vi "RegTester.vi"() -> ()   [LabVIEW 2012]
uses:
  <vilib>/Utility/file.llb/Write To Spreadsheet File (DBL).vi
  <vilib>/vision/NI_Vision_Development_Module.lvlib
panel:
  out "alignment quality":dbl[](graph)
  out "x translation":dbl[](graph)
  in  "x translation file":path
  in  "quality array file":path
  out "error out":errorcluster
  in  "Registration parameters":T1={"Sampling Percentage"=0.2, "maximum iteration"=200, "number of bins"=200}
  in  "background":path
  in  "image folder":path
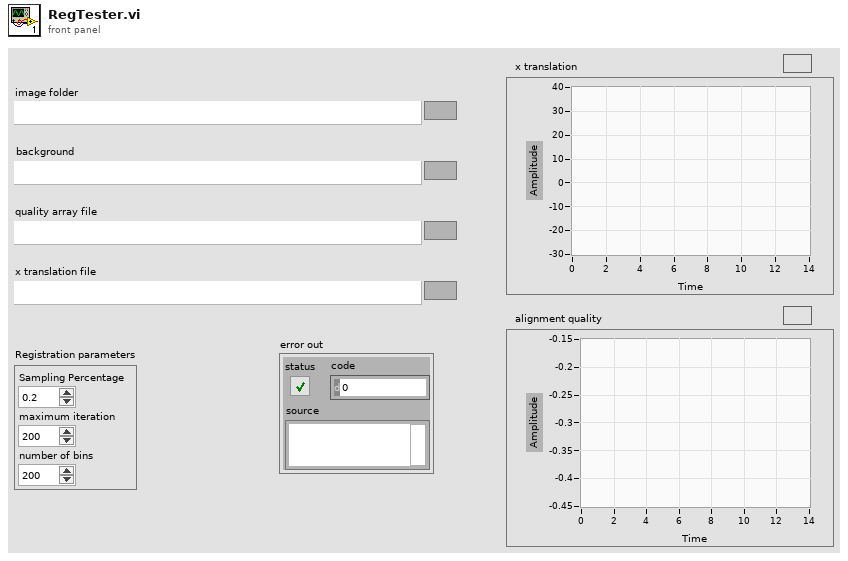
[diagram p1: front panel]
types:
  T1 = cluster{"Sampling Percentage":dbl, "maximum iteration":i32, "number of bins":u32}
  T2 = typedef "Image Type" = u32
  T3 = typedef "IMAQ Image.ctl" = refnum<image>
  T4 = typedef "ROI Descriptor" = cluster{"Global Rectangle":i32[], "Contours":cluster{"ID":enum32{"External", "Internal"}, "Type":u32, "Coordinates":i32[]}[]}
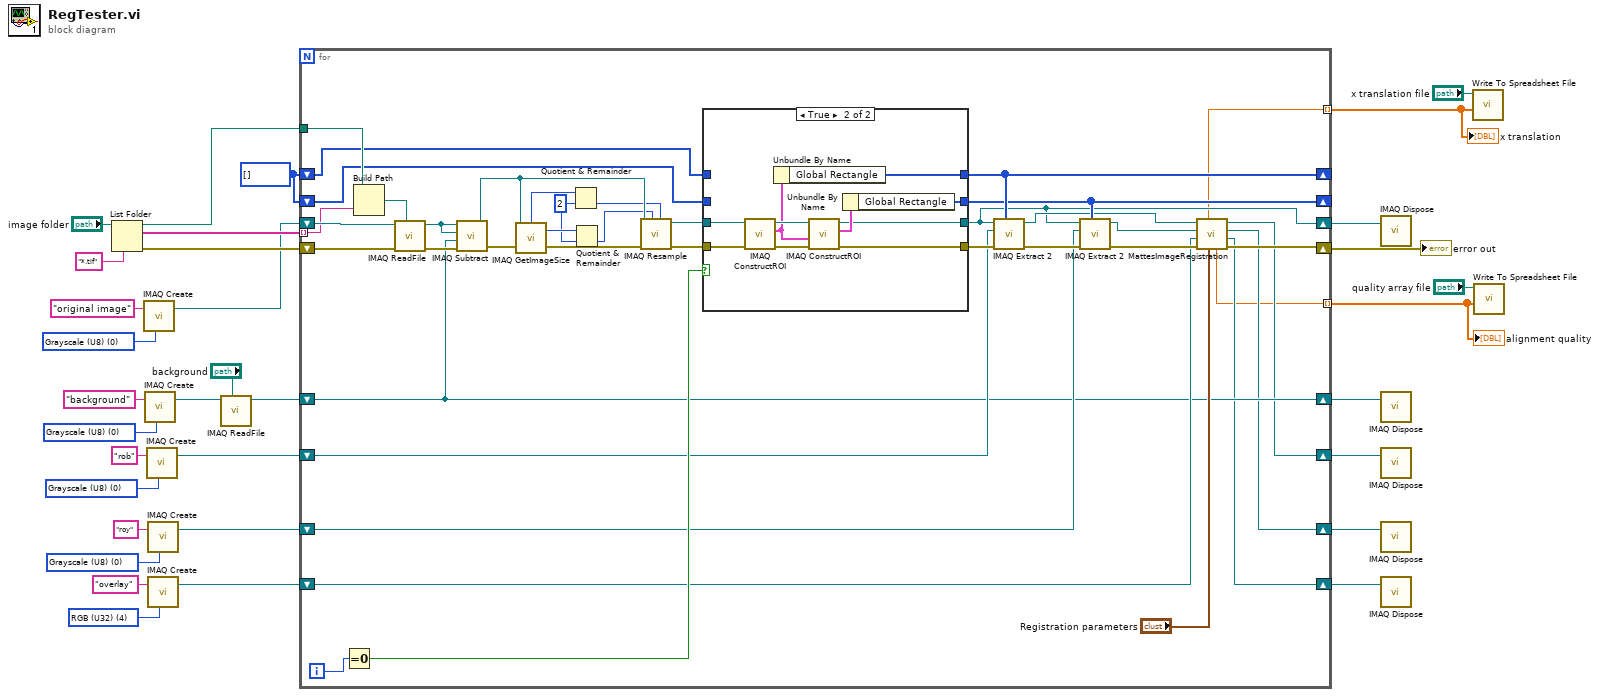
[diagram p0: block diagram]
diagram:
  w14 = i32[] [] ("Global Rectangle")
  w20 = T2 4 items=["Grayscale (U8)", "Grayscale (I16)", "Grayscale (SGL)", "Complex (CSG)", "RGB (U32)", "HSL (U32)", "RGB (U64)", "Grayscale (U16)"] ("Image Type")
  w22 = T2 0 items=["Grayscale (U8)", "Grayscale (I16)", "Grayscale (SGL)", "Complex (CSG)", "RGB (U32)", "HSL (U32)", "RGB (U64)", "Grayscale (U16)"] ("Image Type")
  w23 = T2 0 items=["Grayscale (U8)", "Grayscale (I16)", "Grayscale (SGL)", "Complex (CSG)", "RGB (U32)", "HSL (U32)", "RGB (U64)", "Grayscale (U16)"] ("Image Type")
  w24 = T2 0 items=["Grayscale (U8)", "Grayscale (I16)", "Grayscale (SGL)", "Complex (CSG)", "RGB (U32)", "HSL (U32)", "RGB (U64)", "Grayscale (U16)"] ("Image Type")
  w25 = T2 0 items=["Grayscale (U8)", "Grayscale (I16)", "Grayscale (SGL)", "Complex (CSG)", "RGB (U32)", "HSL (U32)", "RGB (U64)", "Grayscale (U16)"] ("Image Type")
  n1 = List Folder(path="image folder", pattern="*.tif") -> (path out=w16:path, filenames=w27:string[], error out=w26:errorcluster)  [unwired: 2 in, 1 out]
  n2 = call "IMAQ Create"("Image Name"="original image", "Image Type"=w25) -> ("New Image"=w17:T3)  [unwired: 3 in, 1 out]
  n3 = call "IMAQ Create"("Image Name"="background", "Image Type"=w24) -> ("New Image"=w19:T3)  [unwired: 3 in, 1 out]
  n4 = call "IMAQ Create"("Image Name"="rob", "Image Type"=w23) -> ("New Image"=w13:T3)  [unwired: 3 in, 1 out]
  n5 = call "IMAQ Create"("Image Name"="roy", "Image Type"=w22) -> ("New Image"=w12:T3)  [unwired: 3 in, 1 out]
  n6 = call "IMAQ Create"("Image Name"="overlay", "Image Type"=w20) -> ("New Image"=w11:T3)  [unwired: 3 in, 1 out]
  n7 = call "IMAQ ReadFile"("File Path"="background", "Image"=w19) -> ("Image Out"=w15:T3)  [unwired: 5 in, 4 out]
  n8 = for {
    tunnel: w27 -> [w70] mode=indexing
    shift-right: [w42] -> w5
    shift-left: w26 -> [w73]
    shift-right: [w41] -> w10
    shift-left: w17 -> [w72]
    tunnel: w16 -> [w71]
    shift-right: [w51] -> _
    shift-left: w14 -> [w54]
    shift-right: [w48] -> _
    shift-left: w14 -> [w55]
    shift-right: [w40] -> w9
    shift-left: w15 -> [w40]
    shift-right: [w39] -> w8
    shift-left: w13 -> [w52]
    shift-right: [w38] -> w7
    shift-left: w12 -> [w49]
    shift-right: [w37] -> w6
    shift-left: w11 -> [w46]
    tunnel: [w36] -> w2 mode=indexing
    tunnel: [w35] -> w1 mode=indexing
    i -> [w67]
    w62 = 2 ("y")
    n9 = Equal To 0?(x=w67) -> (x = 0?=w66:bool)
    n10 = Build Path(base path=w71, name or relative path=w70) -> (appended path=w69:path)
    n11 = call "IMAQ ReadFile"("File Path"=w69, "error in (no error)"=w73, "Image"=w72) -> ("error out"=w68:errorcluster, "Image Out"=w34:T3)  [unwired: 4 in, 3 out]
    n12 = call "IMAQ Subtract"("Image Src A"=w34, "Image Dst"=w34, "Image Src B"=w40, "error in (no error)"=w68) -> ("Image Dst Out"=w61:T3, "error out"=w65:errorcluster)  [unwired: 3 in]
    n13 = call "IMAQ GetImageSize"("Image"=w61, "error in (no error)"=w65) -> ("Y Resolution"=w63:i32, "X Resolution"=w64:i32, "error out"=w59:errorcluster)  [unwired: 2 in]
    n14 = Quotient & Remainder(x=w64, y=w62) -> (floor(x/y)=w56:i32)  [unwired: 1 out]
    n15 = Quotient & Remainder(x=w63, y=w62) -> (floor(x/y)=w57:i32)  [unwired: 1 out]
    n16 = call "IMAQ Resample"("X Resolution"=w56, "Y Resolution"=w57, "error in (no error)"=w59, "Image Src"=w61) -> ("error out"=w58:errorcluster, "Image Dst Out"=w60:T3)  [unwired: 6 in]
    n17 = case shown="True" w66 {
      tunnel: w58 -> [w75 w87]
      tunnel: w60 -> [w76 w86]
      tunnel: [w75 w81] -> w53
      tunnel: [w76 w80] -> w41
      tunnel: [w77 w79] -> w48
      tunnel: [w74 w78] -> w51
      tunnel: w55 -> [w77 _]
      tunnel: w54 -> [w74 _]
      frame False {
      }
      frame True {
        n18 = call "IMAQ ConstructROI"("error in (no error)"=w87, "Image"=w86) -> ("error out"=w84:errorcluster, "ROI Descriptor Out"=w83:T4, "Image Out (duplicate)"=w85:T3)  [unwired: 6 in, 1 out]
        n19 = Unbundle By Name(w83) -> ("Global Rectangle"=w78:i32[])
        n20 = call "IMAQ ConstructROI"("error in (no error)"=w84, "ROI Descriptor In (None)"=w83, "Image"=w85) -> ("error out"=w81:errorcluster, "ROI Descriptor Out"=w82:T4, "Image Out (duplicate)"=w80:T3)  [unwired: 5 in, 1 out]
        n21 = Unbundle By Name(w82) -> ("Global Rectangle"=w79:i32[])
      }
    }
    n22 = call "IMAQ Extract 2"("Optional Rectangle"=w51, "error in (no error)"=w53, "Image Dst"=w52, "Image Src"=w41) -> ("error out"=w50:errorcluster, "Image Dst Out"=w45:T3)  [unwired: 6 in]
    n23 = call "IMAQ Extract 2"("Optional Rectangle"=w48, "error in (no error)"=w50, "Image Dst"=w49, "Image Src"=w41) -> ("error out"=w47:errorcluster, "Image Dst Out"=w44:T3)  [unwired: 6 in]
    n24 = call "MattesImageRegistration.vi"("Registration parameters"="Registration parameters", "error in (no error)"=w47, "False color image in"=w46, "Moving image in"=w44, "Fixed image in"=w45) -> ("error out"=w42:errorcluster, "False color alignment image"=w37:T3, "Moving image out (duplicate)"=w38:T3, "Fixed image out (duplicate)"=w39:T3, "alignment quality"=w35:dbl, "x translation"=w36:dbl)  [unwired: 1 out]
  }
  "error out" <- w5
  "x translation" <- w2
  "alignment quality" <- w1
  n25 = call "IMAQ Dispose"("Image"=w10) -> ()  [unwired: 5 in, 1 out]
  n26 = call "IMAQ Dispose"("Image"=w9) -> ()  [unwired: 5 in, 1 out]
  n27 = call "IMAQ Dispose"("Image"=w8) -> ()  [unwired: 5 in, 1 out]
  n28 = call "IMAQ Dispose"("Image"=w7) -> ()  [unwired: 5 in, 1 out]
  n29 = call "IMAQ Dispose"("Image"=w6) -> ()  [unwired: 5 in, 1 out]
  n30 = call-poly <vilib>:"Write To Spreadsheet File.vi"("1D data"=w2, "file path (dialog if empty)"="x translation file") -> ()  [unwired: 6 in, 1 out]
  n31 = call-poly <vilib>:"Write To Spreadsheet File.vi"("1D data"=w1, "file path (dialog if empty)"="quality array file") -> ()  [unwired: 6 in, 1 out]
